vi "Keys Example.vi"() -> ()   [LabVIEW 2019, in "Redis Client Examples.lvlib"]
uses:
  Redis Client Examples.lvlib
  lib/RESP3-for-LabVIEW/RESP3/types/RESP3 Type.ctl
  353d0c99-d3b3-4edc-b1af-40a4faf80560.vi
  Redis Client for LabVIEW/Redis Pipelining TCP Client/Redis Pipelining TCP Client.lvclass
  C:/Users/Nicholas Folse/Documents/workspace/github-tauterra.llc/Redis Client for LabVIEW/Redis Client for LabVIEW/Redis Client/Redis Client.lvclass
  RESP3 for LabVIEW/RESP3/high-level/RESP3 Get String.vi
  Redis Client for LabVIEW/Redis Client/Redis Client.lvclass
  lib/RESP3-for-LabVIEW/RESP3/RESP3.lvlib
panel:
  out "random key":string
  out "PTTL":i64
  out "# exists":i64
  out "serialized value":string
  out "DEL result":variant
  in  "value":string="Hello"
  out "is null?":bool=TRUE
  out "actual RESP3 type":T1
  out "error out":errorcluster
  in  "options":T2={"ms timeout"=-1, "expire time"=timestamp(0 s since 1904-01-01), "NX"=FALSE, "XX"=FALSE, "KEEPTTL"=FALSE, "GET"=FALSE}
  in  "milliseconds to wait":u32
  out "response":variant
  out "String out":string
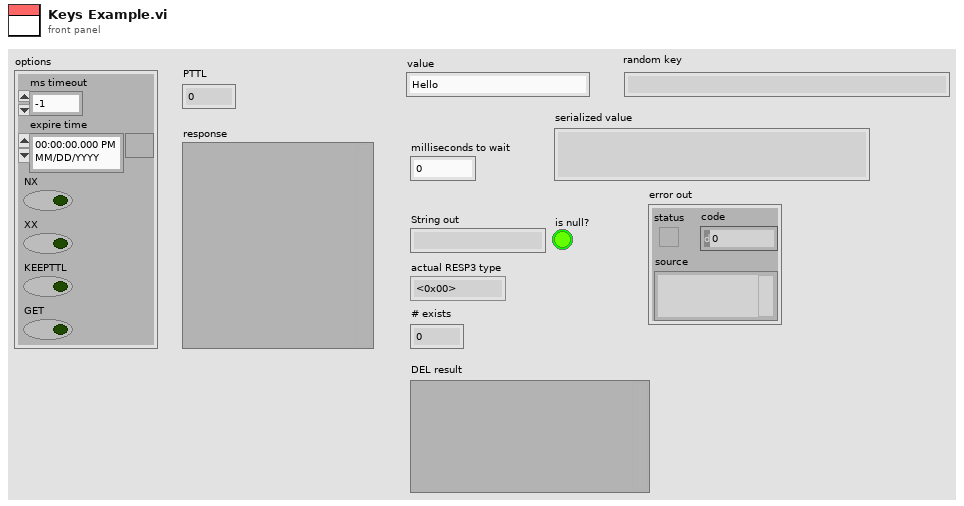
[diagram p1: front panel]
types:
  T1 = typedef "RESP3.lvlib/RESP3 Type.ctl" = enum8{"<0x00>", "<0x01>", "<0x02>", "<0x03>", "<0x04>", "<0x05>", "<0x06>", "<0x07>", "<0x08>", "<0x09>", "<0x0A>", "<0x0B>", "<0x0C>", "<0x0D>", "<0x0E>", "<0x0F>", "<0x10>", "<0x11>", "<0x12>", "<0x13>", "<0x14>", "<0x15>", "<0x16>", "<0x17>", "<0x18>", "<0x19>", "<0x1A>", "<0x1B>", "<0x1C>", "<0x1D>", "<0x1E>", "<0x1F>", "\" \"", "BLOB ERROR", "\"\"\"", "BOOLEAN", "BLOB", "MAP", "\"&\"", "\"'\"", "BIG NUMBER", "\")\"", "ARRAY", "STRING", "DOUBLE", "ERROR", "END", "\"/\"", "\"0\"", "\"1\"", "\"2\"", "\"3\"", "\"4\"", "\"5\"", "\"6\"", "\"7\"", "\"8\"", "\"9\"", "INTEGER", "STREAM", "\"<\"", "VERBATIM STRING", "PUSH", "\"?\"", "\"@\"", "\"A\"", "\"B\"", "\"C\"", "\"D\"", "\"E\"", "\"F\"", "\"G\"", "\"H\"", "\"I\"", "\"J\"", "\"K\"", "\"L\"", "\"M\"", "\"N\"", "\"O\"", "\"P\"", "\"Q\"", "\"R\"", "\"S\"", "\"T\"", "\"U\"", "\"V\"", "\"W\"", "\"X\"", "\"Y\"", "\"Z\"", "\"[\"", "\"\\\"", "\"]\"", "\"^\"", "NULL", "\"`\"", "\"a\"", "\"b\"", "\"c\"", "\"d\"", "\"e\"", "\"f\"", "\"g\"", "\"h\"", "\"i\"", "\"j\"", "\"k\"", "\"l\"", "\"m\"", "\"n\"", "\"o\"", "\"p\"", "\"q\"", "\"r\"", "\"s\"", "\"t\"", "\"u\"", "\"v\"", "\"w\"", "\"x\"", "\"y\"", "\"z\"", "\"{\"", "ATTRIBUTES", "\"}\"", "SET", "<0x7F>", "<0x80>", "<0x81>", "<0x82>", "<0x83>", "<0x84>", "<0x85>", "<0x86>", "<0x87>", "<0x88>", "<0x89>", "<0x8A>", "<0x8B>", "<0x8C>", "<0x8D>", "<0x8E>", "<0x8F>", "<0x90>", "<0x91>", "<0x92>", "<0x93>", "<0x94>", "<0x95>", "<0x96>", "<0x97>", "<0x98>", "<0x99>", "<0x9A>", "<0x9B>", "<0x9C>", "<0x9D>", "<0x9E>", "<0x9F>", "<0xA0>", "<0xA1>", "<0xA2>", "<0xA3>", "<0xA4>", "<0xA5>", "<0xA6>", "<0xA7>", "<0xA8>", "<0xA9>", "<0xAA>", "<0xAB>", "<0xAC>", "<0xAD>", "<0xAE>", "<0xAF>", "<0xB0>", "<0xB1>", "<0xB2>", "<0xB3>", "<0xB4>", "<0xB5>", "<0xB6>", "<0xB7>", "<0xB8>", "<0xB9>", "<0xBA>", "<0xBB>", "<0xBC>", "<0xBD>", "<0xBE>", "<0xBF>", "<0xC0>", "<0xC1>", "<0xC2>", "<0xC3>", "<0xC4>", "<0xC5>", "<0xC6>", "<0xC7>", "<0xC8>", "<0xC9>", "<0xCA>", "<0xCB>", "<0xCC>", "<0xCD>", "<0xCE>", "<0xCF>", "<0xD0>", "<0xD1>", "<0xD2>", "<0xD3>", "<0xD4>", "<0xD5>", "<0xD6>", "<0xD7>", "<0xD8>", "<0xD9>", "<0xDA>", "<0xDB>", "<0xDC>", "<0xDD>", "<0xDE>", "<0xDF>", "<0xE0>", "<0xE1>", "<0xE2>", "<0xE3>", "<0xE4>", "<0xE5>", "<0xE6>", "<0xE7>", "<0xE8>", "<0xE9>", "<0xEA>", "<0xEB>", "<0xEC>", "<0xED>", "<0xEE>", "<0xEF>", "<0xF0>", "<0xF1>", "<0xF2>", "<0xF3>", "<0xF4>", "<0xF5>", "<0xF6>", "<0xF7>", "<0xF8>", "<0xF9>", "<0xFA>", "<0xFB>", "<0xFC>", "<0xFD>", "<0xFE>"}
  T2 = cluster{"ms timeout":i64, "expire time":timestamp, "NX":bool, "XX":bool, "KEEPTTL":bool, "GET":bool}
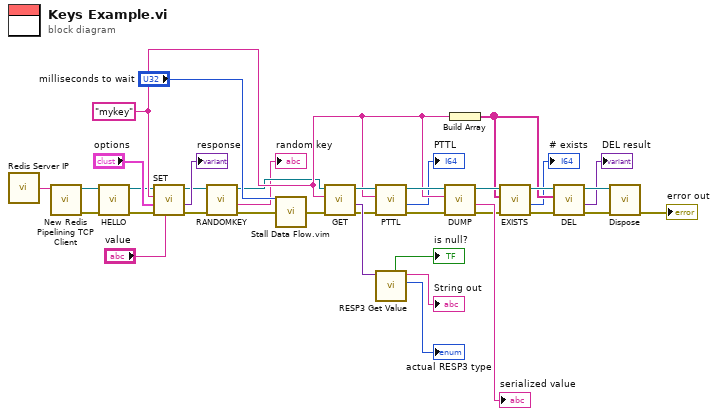
[diagram p0: block diagram]
diagram:
  w11 = "mykey" ("key")
  n1 = call "Redis Server IP.vi"() -> ("server IP"=w36:string)
  n2 = call "New Redis Pipelining TCP Client.vi"("address"=w36) -> ("error out"=w7:errorcluster, "Redis Pipelining TCP Client out"=w10:refnum<class "Redis Pipelining TCP Client.lvclass">)  [unwired: 9 in]
  n3 = call "HELLO.vi"("error in (no error)"=w7, "Redis Client in"=w10) -> ("error out"=w8:errorcluster, "Redis Client out"=w9:refnum<class "Redis Pipelining TCP Client.lvclass">)  [unwired: 7 in, 1 out]
  n4 = call "SET.vi"("value"="value", "error in (no error)"=w8, "options"="options", "key"=w11, "Redis Client in"=w9) -> ("error out"=w4:errorcluster, "response"=→"response":variant, "Redis Client out"=w5:refnum<class "Redis Pipelining TCP Client.lvclass">)  [unwired: 4 in]
  n5 = call "RANDOMKEY.vi"("error in (no error)"=w4, "Redis Client in"=w5) -> ("error out"=w3:errorcluster, "random key"=→"random key":string, "Redis Client out"=w2:refnum<class "Redis Pipelining TCP Client.lvclass">)  [unwired: 6 in, 1 out]
  n6 = call "Stall Data Flow.vim"("value in"=w3, "milliseconds to wait"="milliseconds to wait") -> ("value out"=w33:errorcluster)  [unwired: 1 out]
  n7 = call "GET.vi"("error in (no error)"=w33, "key"=w11, "Redis Client in"=w2) -> ("error out"=w12:errorcluster, "value"=w16:variant, "Redis Client out"=w15:refnum<class "Redis Pipelining TCP Client.lvclass">)  [unwired: 5 in, 1 out]
  n8 = call "PTTL.vi"("error in (no error)"=w12, "key"=w11, "Redis Client in"=w15) -> ("error out"=w13:errorcluster, "PTTL"=→"PTTL":i64, "Redis Client out"=w14:refnum<class "Redis Pipelining TCP Client.lvclass">)  [unwired: 6 in]
  n9 = call-poly "RESP3 Get Value.vi"("RESP3 Value in"=w16) -> ("actual RESP3 type"=→"actual RESP3 type":T1, "String out"=→"String out":string, "is null?"=→"is null?":bool)  [unwired: 7 in, 1 out]
  n10 = call "DUMP.vi"("error in (no error)"=w13, "key"=w11, "Redis Client in"=w14) -> ("error out"=w21:errorcluster, "serialized value"=→"serialized value":string, "Redis Client out"=w22:refnum<class "Redis Pipelining TCP Client.lvclass">)  [unwired: 5 in, 1 out]
  n11 = Build Array(w11) -> (w18:string[])
  n12 = call "EXISTS.vi"("error in (no error)"=w21, "keys"=w18, "Redis Client in"=w22) -> ("error out"=w20:errorcluster, "# exists"=→"# exists":i64, "Redis Client out"=w19:refnum<class "Redis Pipelining TCP Client.lvclass">)  [unwired: 6 in]
  n13 = call "DEL.vi"("error in (no error)"=w20, "keys"=w18, "Redis Client in"=w19) -> ("error out"=w26:errorcluster, "value"=→"DEL result":variant, "Redis Client out"=w25:refnum<class "Redis Pipelining TCP Client.lvclass">)  [unwired: 6 in]
  n14 = call-dynamic "Dispose.vi"("error in (no error)"=w26, "Redis Pipelining TCP Client in"=w25) -> ("error out"=→"error out":errorcluster)  [unwired: 9 in]
